vi "ProdaNG.Example.GetLanguages.vi"() -> ()   [LabVIEW 2016]
panel:
  out "error out":errorcluster {"code" format="%.2f"}
  out "Languages":string[](array[string])
  in  "Connection string":string="lcptb/lcptb@proda_wpl_dev"
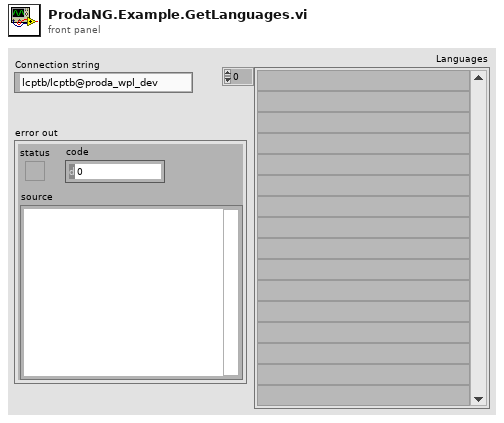
[diagram p1: front panel]
types:
  T1 = typedef "ProdaNG.Language.ctl" = cluster{"i_id":i32, "isoCode":string, "name":string}
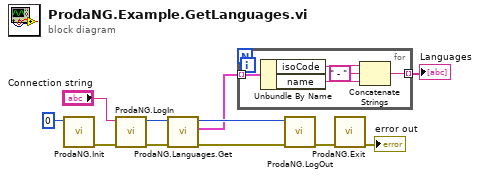
[diagram p0: block diagram]
diagram:
  n1 = call "ProdaNG.Init.vi"("numContexts (0: unlimited)"=0 ("numContexts")) -> ("error out"=w11:errorcluster)  [unwired: 10 in]
  n2 = call "ProdaNG.LogIn.vi"("error in"=w11, "ConnectionString"="Connection string") -> ("error out"=w7:errorcluster, "dbHandle"=w6:i32)  [unwired: 7 in, 1 out]
  n3 = call "ProdaNG.Languages.Get.vi"("error in (no error)"=w7, "dbHandleIn"=w6) -> ("error out"=w5:errorcluster, "Languages"=w3:T1[], "dbHandle"=w4:i32)  [unwired: 7 in]
  n4 = for {
    tunnel: w3 -> [w16] mode=indexing
    tunnel: [w14] -> w2 mode=indexing
    n5 = Unbundle By Name(w16) -> ("isoCode"=w13:string, "name"=w15:string)
    n6 = Concatenate Strings(w13, " - " ("string"), w15) -> (w14:string)
  }
  "Languages" <- w2
  n7 = call "ProdaNG.LogOut.vi"("error in"=w5, "dbHandleIn"=w4) -> ("error out"=w9:errorcluster)  [unwired: 9 in]
  n8 = call "ProdaNG.Exit.vi"("error in (no error)"=w9) -> ("error out"=→"error out":errorcluster)  [unwired: 10 in]
